vi "Lab1(Ver3).vi"() -> ()   [LabVIEW 2010]
uses:
  <vilib>/measure/maspectr.llb/FFT Spectrum (Mag-Phase) for 1 Chan.vi
  <vilib>/measure/NI_MABase.lvlib
  <vilib>/measure/NI_MAPro.lvlib
  <vilib>/ptbypt/NI_PtbyPt.lvlib
panel:
  out "power ratio":dbl
  in  "stop":bool
  out "baseband signal (time-domain)":waveform(dbl)(graph)
  out "baseband signal (frequency-domain)":cluster{"f0":dbl, "df":dbl, "magnitude":dbl[]}(graph)
  out "modulated signal (frequency-domain)":cluster{"f0":dbl, "df":dbl, "magnitude":dbl[]}(graph)
  out "modulated signal (time-domain)":waveform(dbl)(graph)
  in  "mod index":dbl(slide)=1.0 scale=0.0..1.0
  in  "modulation frequency":dbl(knob)=10.0 scale=0.0..1000.0
  in  "carrier frequency":dbl(knob)=10.0 scale=0.0..500000.0
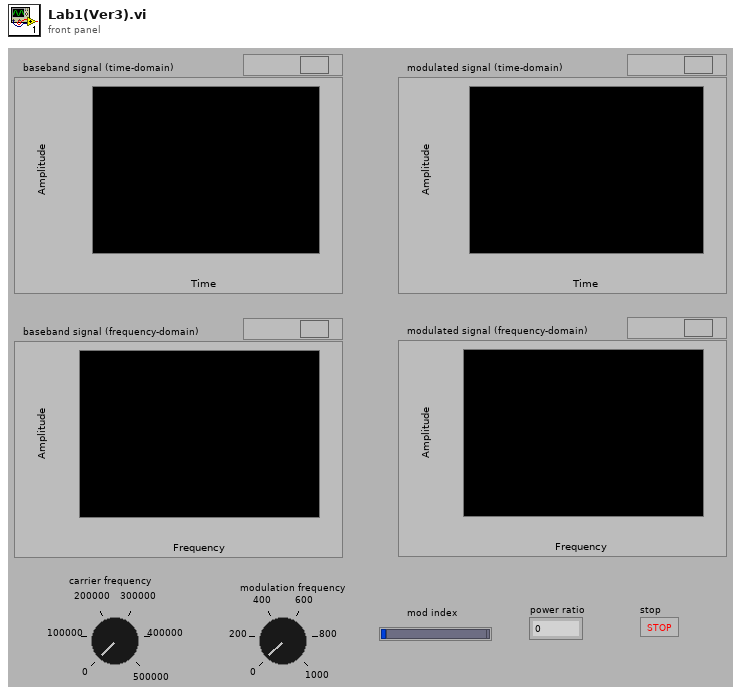
[diagram p1: front panel]
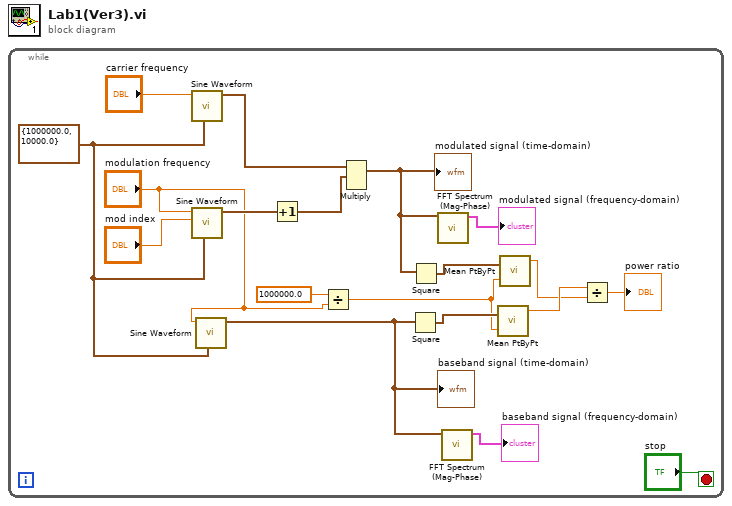
[diagram p0: block diagram]
diagram:
  n1 = while {
    stop <- "stop" stop-if-true
    w1 = cluster{"Fs":dbl, "#s":dbl} {"Fs"=1000000.0, "#s"=10000.0} ("sampling info")
    n2 = call <vilib>:"Sine Waveform.vi"("sampling info"=w1, "frequency"="carrier frequency") -> ("signal out"=w17:waveform(dbl))  [unwired: 8 in, 1 out]
    n3 = call <vilib>:"Sine Waveform.vi"("sampling info"=w1, "amplitude"="mod index", "frequency"="modulation frequency") -> ("signal out"=w6:waveform(dbl))  [unwired: 7 in, 1 out]
    n4 = call <vilib>:"Sine Waveform.vi"("sampling info"=w1, "frequency"="modulation frequency") -> ("signal out"=w3:waveform(dbl))  [unwired: 8 in, 1 out]
    "baseband signal (time-domain)" <- w3
    n5 = Increment(x=w6) -> (x+1=w16:waveform(dbl))
    n6 = Divide(x=1000000.0, y="modulation frequency") -> (x/y=w8:dbl)
    n7 = Multiply(1:w16, 2:w17) -> (0:w12:waveform(dbl))  [unwired: 1 in, 1 out]
    "modulated signal (time-domain)" <- w12
    n8 = Square(x=w3) -> (x^2=w11:waveform(dbl))
    n9 = Square(x=w12) -> (x^2=w10:waveform(dbl))
    n10 = call-poly <vilib>:"FFT Spectrum (Mag-Phase).vi"("time signal"=w12) -> ("magnitude"=→"modulated signal (frequency-domain)":cluster{"f0":dbl, "df":dbl, "magnitude":dbl[]})  [unwired: 6 in, 4 out]
    n11 = call-poly <vilib>:"FFT Spectrum (Mag-Phase).vi"("time signal"=w3) -> ("magnitude"=→"baseband signal (frequency-domain)":cluster{"f0":dbl, "df":dbl, "magnitude":dbl[]})  [unwired: 6 in, 4 out]
    n12 = call <vilib>:"Mean PtByPt.vi"("x"=w11, "sample length"=w8) -> ("mean"=w5:dbl)  [unwired: 2 in, 1 out]
    n13 = call <vilib>:"Mean PtByPt.vi"("x"=w10, "sample length"=w8) -> ("mean"=w4:dbl)  [unwired: 2 in, 1 out]
    n14 = Divide(x=w5, y=w4) -> (x/y=→"power ratio":dbl)
  }
